vi "Detect Transition to Load.vi"(5 "Main References":T2, 8 "error in (no error)":errorcluster, 10 "Cart Array":bool[](array[boolean])) -> (0 "error out":errorcluster, 3 "Analysis":T1[](array[typedef]))   [LabVIEW 2020]
uses:
  Main Refs.ctl
  Hardware/Tecan/Pump Config.ctl
  Timing Specs.ctl
  Vacuum Specs.ctl
  Cartridges.ctl
  Cartridge Status.ctl
  Commands.ctl
  Lib/Time/Wells.ctl
  Lib/Time/Bottles.ctl
  Process State.ctl
  Vacuum Test.ctl
  Hardware/Mot Stage Mngr.ctl
  Hardware/16CH Denkovi Mngr.ctl
  Hardware/DAQ Mngr.ctl
panel:
  # "Tecan Pump"
  # "Pressure"
  # "General"
  # "Timing"
  # "Protocol"
  # "Zaber"
  # "NFC Reader 1"
  # "NFC  Reader 2"
  # "NFC Reader 3"
  # "NFC Reader 4"
  # "System"
  # "Cartridge Utitlies"
  # "Wells"
  # "times"
  # "from"
  # "State Machine"
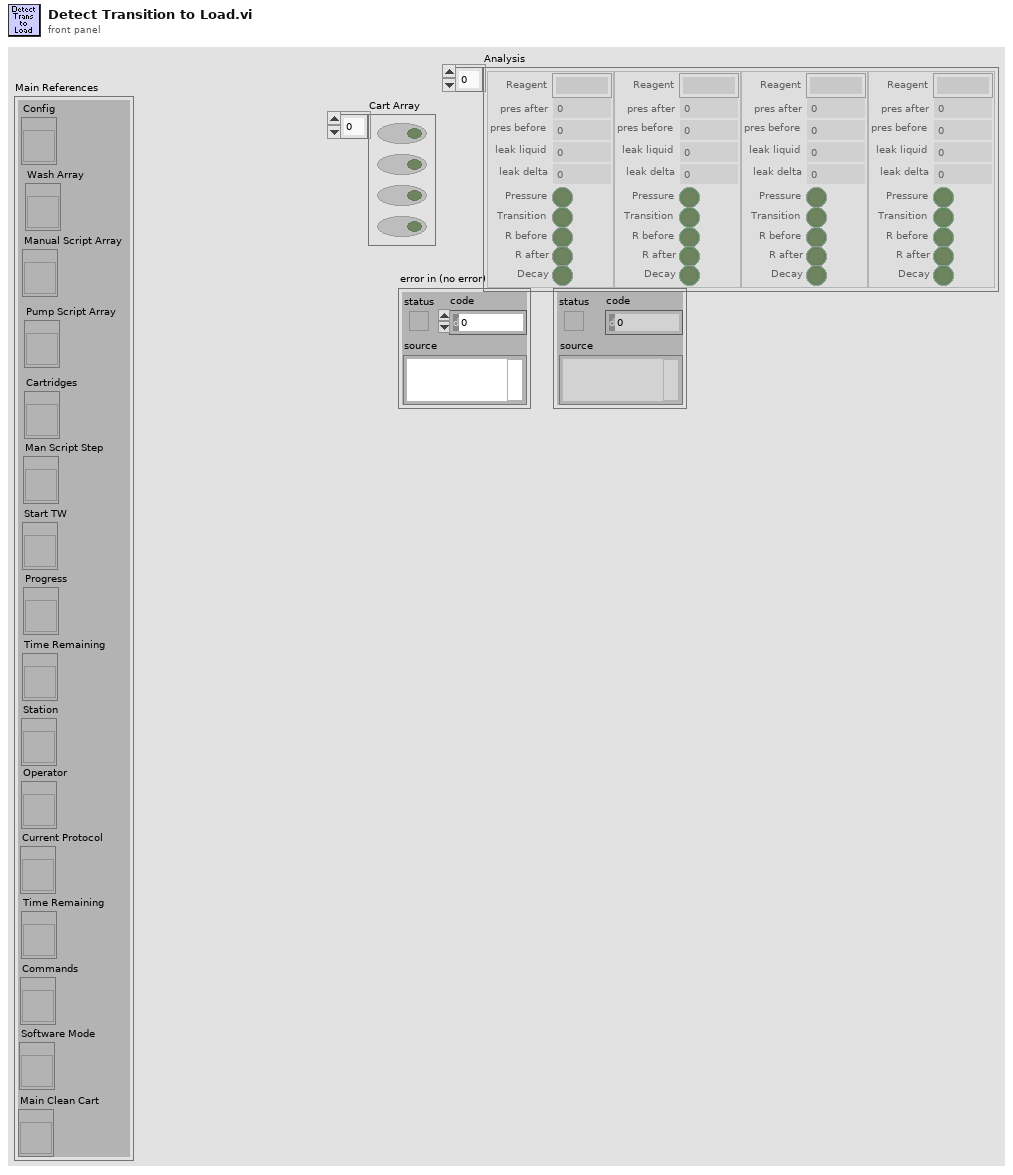
[diagram p1: front panel]
types:
  T1 = typedef "Vacuum Test.ctl" = cluster{"pres after":dbl, "pres before":dbl, "leak liquid":dbl, "leak delta":dbl, "Transition":bool, "Pressure":bool, "R before":bool, "R after":bool, "Reagent":string, "Decay":bool}
  T2 = typedef "Main Refs.ctl" = cluster{"Config":refnum<vi>, "Wash Array":refnum<vi>, "Manual Script Array":refnum<vi>, "Pump Script Array":refnum<vi>, "Cartridges":refnum<vi>, "Man Script Step":refnum<vi>, "Start TW":refnum<vi>, "Progress":refnum<vi>, "Time Remaining":refnum<vi>, "Station":refnum<vi>, "Operator":refnum<vi>, "Current Protocol":refnum<vi>, "Time Remaining":refnum<vi>, "Commands":refnum<vi>, "Software Mode":refnum<vi>, "Main Clean Cart":refnum<vi>}
  T3 = typedef "16CH Denkovi Mngr.ctl" = enum16{"Search", "Init", "Set Peristaltic", "Set Pressure", "Set Vacuum", "Pres Vent&Close", "Vac Vent&Close", "Pres ON", "Vac ON", "Set All Relays", "Set One Relay", "Read Relays", "Close"}
  T4 = typedef "DAQ Mngr.ctl" = enum16{"Init", "Read Pressure", "Read Vacuum", "Analyze Pressure", "Analyze Vacuum", "Read Cartridges", "Lock Cartridge", "Unlock Cartridge", "Read PS", "Pinch Valve Engage", "Pinch Valve Disengage", "Close"}
  T5 = typedef "Mot Stage Mngr.ctl" = enum16{"Connect", "Init", "Status", "Send Cmd", "Current Pos", "Set Accel", "Set Max Vel", "Home", "Rel Move", "Abs Move", "Close"}
  T6 = typedef "Pump Config.ctl" = cluster{"Syringe size":u32, "Syringe address":u32, "# of ports":u32, "Init String":string, "Full Stroke (cnts)":i32, "Model":enum16{"XC", "Centris"}, "TW Position":dbl, "Load Position":dbl, "Bottom Position":dbl, "Station ID":string, "Default Protocol":path, "Dry Time(s)":dbl, "Python Version":string, "NFC SN Array":string[], "Timing":T7, "Pressure Specs":T8}
  T7 = typedef "Timing Specs.ctl" = cluster{"Checking pres and leak":dbl, "Priming input lines":dbl, "Rinsing syringe":dbl, "Filling well X w/ X":dbl, "Drain well X":dbl, "Clearing wells and lines":dbl, "Draining wells":dbl, "Rinsing all wells":dbl, "Testing for leaks/clogs":dbl, "Rinsing wells":dbl}
  T8 = typedef "Vacuum Specs.ctl" = cluster{"Pressure max":dbl, "Pressure min":dbl, "Decay delta":dbl, "Pressure time":dbl, "Conf. R":dbl, "LeakRateMax":dbl}
  T9 = typedef "Pressure Output.ctl" = cluster{"Time(s)":dbl, "Pressure":dbl, "Rate":dbl, "R":dbl}
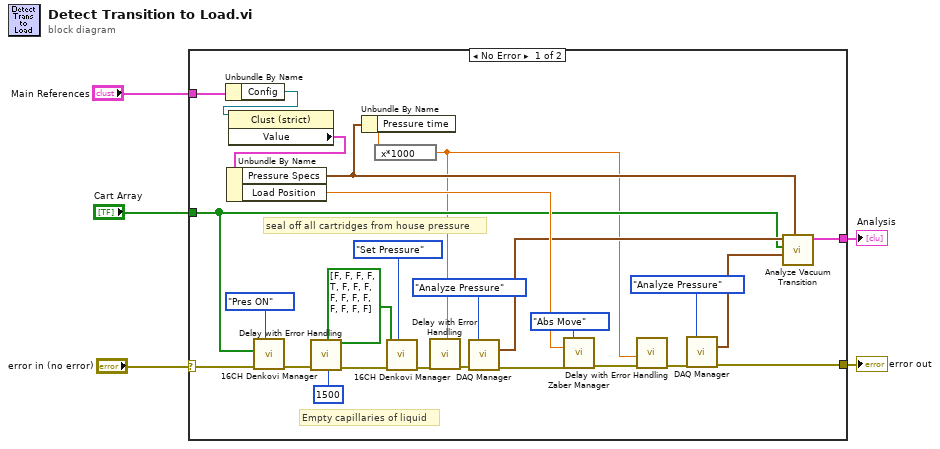
[diagram p0: block diagram]
diagram:
  n1 = case shown="No Error" "error in (no error)" {
    selector: "error in (no error)" -> [w26 w33]
    tunnel: [w17 w33] -> w4
    tunnel: "Cart Array" -> [w15 _]
    tunnel: "Main References" -> [w30 _]
    tunnel: [w16 _] -> w1
    frame No Error {
      # "seal off all cartridges from house pressure"
      # "Empty capillaries of liquid"
      n2 = Unbundle By Name(w30) -> ("Config"=w32:refnum<vi>)
      n3 = property class="Clust (strict)"(reference=w32) -> ("Value"=w29:T6)  [unwired: 1 in, 2 out]
      n4 = Unbundle By Name(w29) -> ("Pressure Specs"=w8:T8, "Load Position"=w28:dbl)
      n5 = call "16CH Denkovi Manager.vi"("Action"=16CH_Denkovi_Mngr."Pres ON", "error in (no error)"=w26, "Relays In"=w15) -> ("error out"=w10:errorcluster)  [unwired: 6 in, 2 out]
      n6 = call "Delay with Error Handling.vi"("error in (no error)"=w10, "Delay (ms)"=u32 1500) -> ("error out"=w9:errorcluster)  [unwired: 9 in]
      n7 = Unbundle By Name(w8) -> ("Pressure time"=w7:dbl)
      n8 = expression code="x*1000"(w7) -> (w6:dbl)
      n9 = call "16CH Denkovi Manager.vi"("Action"=16CH_Denkovi_Mngr."Set Pressure", "error in (no error)"=w9, "Relays In"=bool[] [FALSE, FALSE, FALSE, FALSE, TRUE, FALSE, FALSE, FALSE, FALSE, FALSE, FALSE, FALSE, FALSE, FALSE, FALSE, FALSE]) -> ("error out"=w14:errorcluster)  [unwired: 6 in, 2 out]
      n10 = call "Delay with Error Handling.vi"("error in (no error)"=w14, "Delay (ms)"=w6) -> ("error out"=w25:errorcluster)  [unwired: 9 in]
      n11 = call "DAQ Manager.vi"("DAQ Mngr Action"=DAQ_Mngr."Analyze Pressure", "error in (no error)"=w25) -> ("Pressure Array"=w19:T9[], "error out"=w24:errorcluster)  [unwired: 7 in, 5 out]
      n12 = call "Zaber Manager.vi"("Action"=Mot_Stage_Mngr."Abs Move", "Value"=w28, "error in (no error)"=w24) -> ("error out"=w22:errorcluster)  [unwired: 6 in, 6 out]
      n13 = call "Delay with Error Handling.vi"("error in (no error)"=w22, "Delay (ms)"=w6) -> ("error out"=w21:errorcluster)  [unwired: 9 in]
      n14 = call "DAQ Manager.vi"("DAQ Mngr Action"=DAQ_Mngr."Analyze Pressure", "error in (no error)"=w21) -> ("Pressure Array"=w18:T9[], "error out"=w17:errorcluster)  [unwired: 7 in, 5 out]
      n15 = call "Analyze Vacuum Transition.vi"("Pressure Specs"=w8, "Data After"=w18, "Cart Array"=w15, "Data Before"=w19) -> ("Analysis"=w16:T1[])  [unwired: 5 in, 2 out]
    }
    frame Error {
    }
  }
  "error out" <- w4
  "Analysis" <- w1
